vi "NanoDropDetect.vi"(6 "dB Thresh":dbl, 7 "length":i32, 8 "Max value":dbl, 9 "index":i32, 10 "Array":dbl[][](array[numeric]), 11 "noise":i32) -> (3 "Numeric":i16)   [LabVIEW 2022 SP3]
panel:
  out "Raw data":dbl[][](graph)
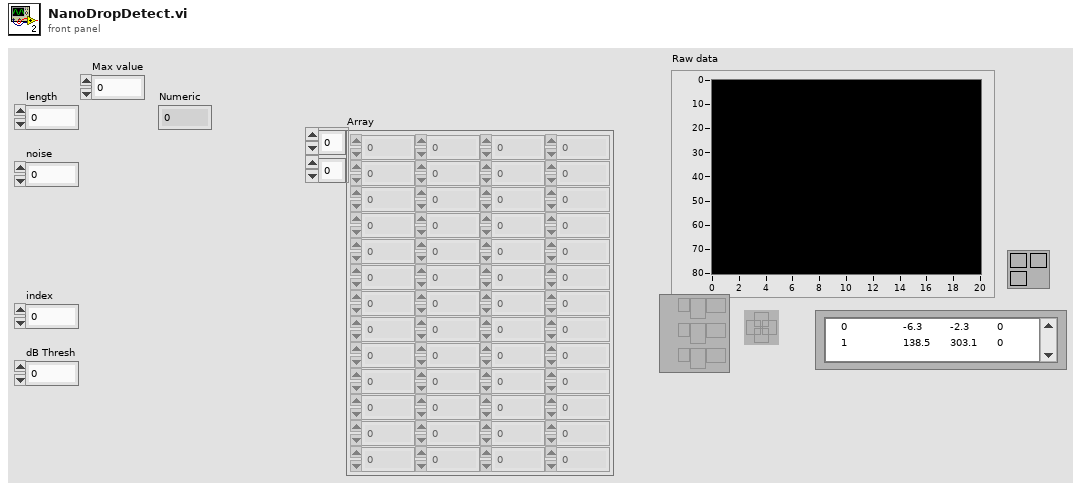
[diagram p1: front panel]
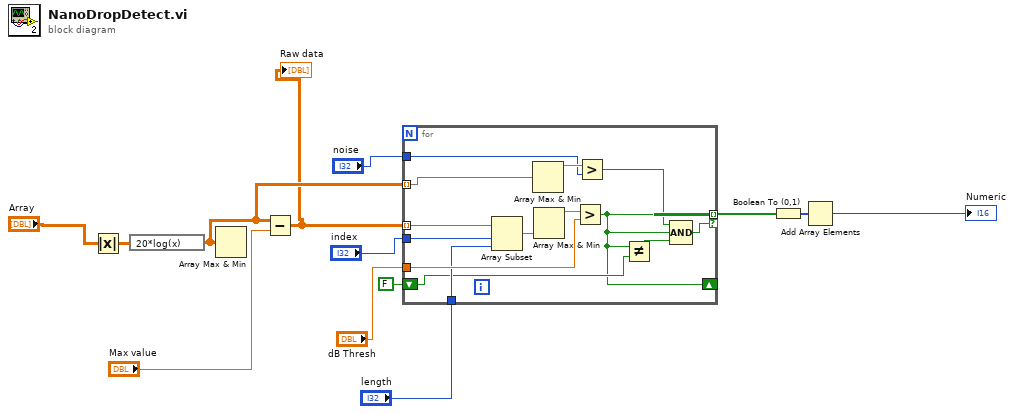
[diagram p0: block diagram]
diagram:
  n1 = Absolute Value(x="Array") -> (abs(x)=w11:dbl[][])
  n2 = expression code="20*log(x)"(w11) -> (w12:dbl[][])
  n3 = Array Max & Min(array=w12) -> ()  [unwired: 4 out]
  n4 = Subtract(x=w12, y="Max value") -> (x-y=w2:dbl[][])
  "Raw data" <- w2
  n5 = for {
    tunnel: w2 -> [w25] mode=indexing
    tunnel: [w14] -> w4 mode=indexing if=w19
    tunnel: "dB Thresh" -> [w26]
    tunnel: "index" -> [w23]
    tunnel: "length" -> [w22]
    shift-right: [w14] -> _
    shift-left: FALSE -> [w21]
    tunnel: w12 -> [w18] mode=indexing
    tunnel: "noise" -> [w15]
    n6 = Array Subset(array=w25, index=w23, length=w22) -> (w24:dbl[])
    n7 = Array Max & Min(array=w18) -> (max value=w17:dbl)  [unwired: 3 out]
    n8 = Array Max & Min(array=w24) -> (max value=w27:dbl)  [unwired: 3 out]
    n9 = Greater?(x=w27, y=w26) -> (0:w14:bool)
    n10 = Greater?(x=w17, y=w15) -> (0:w16:bool)
    n11 = Not Equal?(x=w14, y=w21) -> (x != y?=w20:bool)
    n12 = Compound Arithmetic op=AND(w16, w14, w20) -> (w19:bool)
  }
  n13 = Boolean To (0,1)(Boolean=w4) -> (0, 1=w6:i16[])
  n14 = Add Array Elements(numeric array=w6) -> (sum=→"Numeric":i16)
